vi "Configure Digital Data.vi"(0 "VISA resource name":refnum<visa-resource-name>, 1 "Direction (0: Output)":u16(ring) items=["Output", "Input"], 5 "Data Type (0: Samples)":u16(ring) items=["Samples", "Pre-filtered Samples"], 7 "Word Size (16)":i32=16, 9 "Word Alignment (0: LSB)":u16(ring) items=["LSB", "MSB"], 11 "error in (no error)":errorcluster, 12 "Bit Order (0: LSB)":u16(ring) items=["LSB", "MSB"], 13 "Numeric Format (0: 2's complement)":u16(ring) items=["2's complement", "Offset binary"]) -> (4 "VISA resource name out":refnum<visa-resource-name>, 15 "error out":errorcluster)   [LabVIEW 2011, in "Agilent PSG MXG Series.lvlib"]
doc: "Configures data type, direction, word size, word alignment, bit order and numeric format.\n\n<B>Notes:</B>\n(1) This VI is valid only in E8267D that installs <B>Option 601</B> or <B>Option 602</B> (Internal baseband generator), and <B>Option 003</B> (PSG digital output connectivity with N5102A) or <B>Option 004</B> (PSG digital input connectivity with N5102A)."
uses:
  Agilent PSG MXG Series.lvlib
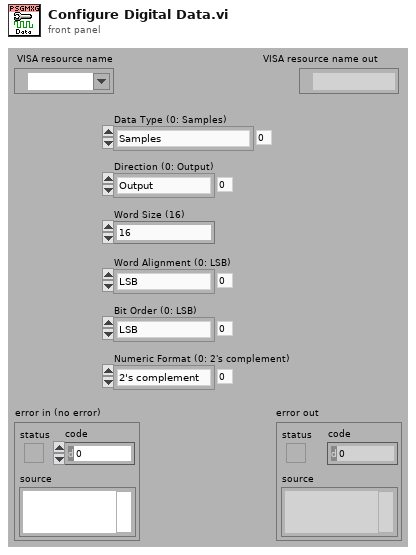
[diagram p1: front panel]
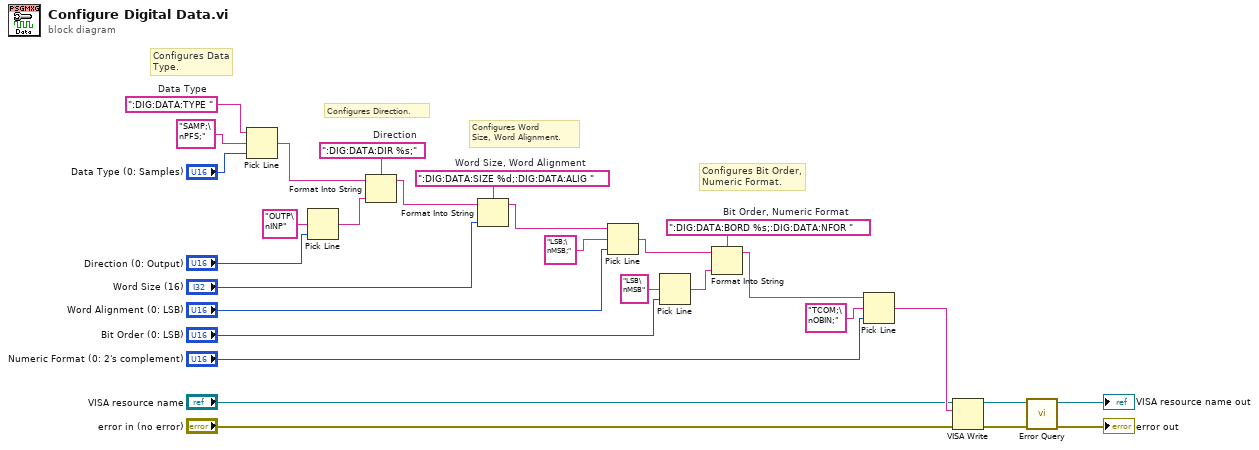
[diagram p0: block diagram]
diagram:
  w15 = ":DIG:DATA:BORD %s;:DIG:DATA:NFOR "  # Bit Order, Numeric Format
  w20 = ":DIG:DATA:SIZE %d;:DIG:DATA:ALIG "  # Word Size, Word Alignment
  w25 = ":DIG:DATA:DIR %s;"  # Direction
  w29 = ":DIG:DATA:TYPE "  # Data Type
  # "Configures Bit Order,\nNumeric Format."
  # "Configures Word\nSize, Word Alignment."
  # "Configures Direction."
  # "Configures Data\nType."
  n1 = Pick Line(string ("")=w29, multi-line string="SAMP;\nPFS;", line index="Data Type (0: Samples)") -> (output string=w26:string)
  n2 = Pick Line(multi-line string="OUTP\nINP", line index="Direction (0: Output)") -> (output string=w22:string)  [unwired: 1 in]
  n3 = Format Into String(format string=w25, initial string=w26, w22) -> (resulting string=w21:string)  [unwired: 1 in, 1 out]
  n4 = Format Into String(format string=w20, initial string=w21, "Word Size (16)") -> (resulting string=w18:string)  [unwired: 1 in, 1 out]
  n5 = Pick Line(string ("")=w18, multi-line string="LSB;\nMSB;", line index="Word Alignment (0: LSB)") -> (output string=w16:string)
  n6 = Pick Line(multi-line string="LSB\nMSB", line index="Bit Order (0: LSB)") -> (output string=w13:string)  [unwired: 1 in]
  n7 = Format Into String(format string=w15, initial string=w16, w13) -> (resulting string=w10:string)  [unwired: 1 in, 1 out]
  n8 = Pick Line(string ("")=w10, multi-line string="TCOM;\nOBIN;", line index="Numeric Format (0: 2's complement)") -> (output string=w7:string)
  n9 = VISA Write(VISA resource name="VISA resource name", write buffer=w7, error in (no error)="error in (no error)") -> (VISA resource name out=w6:refnum<visa-resource-name>, error out=w5:errorcluster)  [unwired: 1 out]
  n10 = call "Error Query.vi"("error in (no error)"=w5, "VISA resource name"=w6) -> ("error out"=→"error out":errorcluster, "VISA resource name out"=→"VISA resource name out":refnum<visa-resource-name>)  [unwired: 6 in, 2 out]
